vi "2022_day01.vi"() -> ()   [LabVIEW 2021]
uses:
  2f9034f6-0eee-4750-bf2c-0a9c5446afb1.vi
  <vilib>/Comparison/Less/Less Functor/Less Functor.lvclass
panel:
  out "Sum of TOP Calories (task 2)":i32
  in  "Sel. TOP cnt":i32=3
  out "TOP Calories":i32[](array[numeric])
  out "max Calories (task 1)":i32
  out "Raw data":i32[](array[numeric])
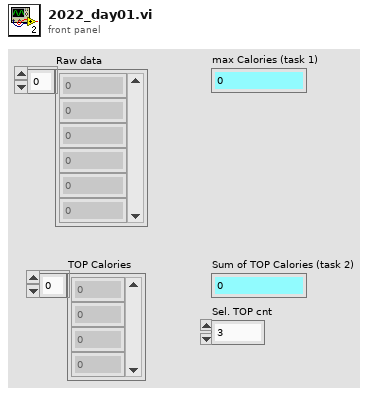
[diagram p1: front panel]
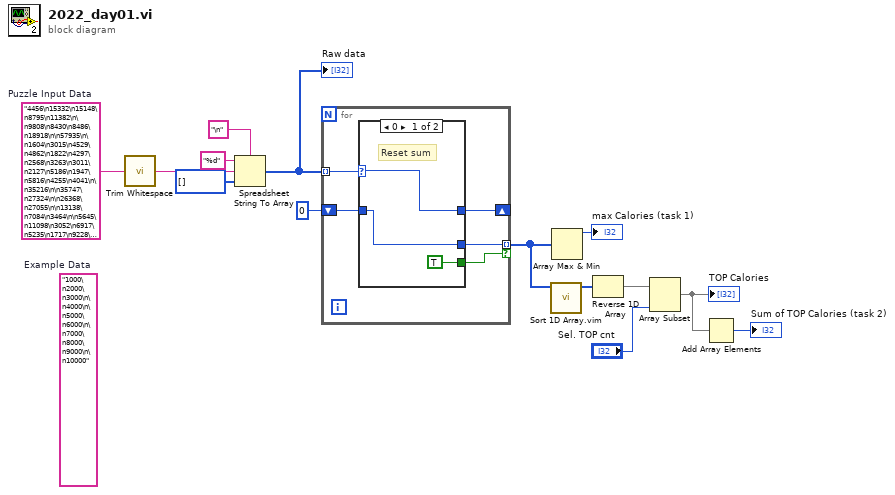
[diagram p0: block diagram]
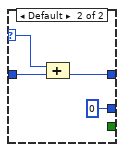
[diagram p2: hidden frame]
diagram:
  (unwired) "1000\n2000\n3000\n\n4000\n\n5000\n6000\n\n7000\n8000\n9000\n\n10000"  # Example Data
  w7 = "4456\n15332\n15148\n8795\n11382\n\n9808\n8430\n8486\n18918\n\n57935\n\n1604\n3015\n4529\n4862\n1822\n4297\n2568\n3263\n3011\n2127\n5186\n1947\n5816\n4255\n4041\n\n35216\n\n35747\n27324\n\n26368\n27055\n\n13138\n7084\n3464\n\n5645\n11098\n3052\n6917\n5235\n1717\n9228\n\n7789\n9290\n5753\n9600\n8631\n6873\n8844\n2228\n5123\n\n5177\n7591\n7973\n2093\n7266\n5307\n3562\n4994\n2681\n2924\n\n15474\n11021\n14987\n18512\n\n12187\n6865\n20315\n\n13751\n\n6467\n8287\n14768\n7194\n9595\n\n3948\n1577\n1989\n\n24800\n23570\n\n2378\n3426\n6782\n7276\n5242\n3067\n4899\n5532\n4877\n6314\n6935\n1956\n\n59761\n\n15344\n4376\n10193\n2616\n4785\n\n2213\n5782\n1524\n5941\n3889\n4619\n5429\n2136\n2728\n3576\n2656\n5164\n4329\n2497\n4708\n\n5683..."  # Puzzle Input Data
  n1 = call <vilib>:"Trim Whitespace.vi"("string"=w7) -> ("trimmed string"=w9:string)  [unwired: 1 in]
  n2 = Spreadsheet String To Array(delimiter (Tab)="\n", format string="%d", spreadsheet string=w9, array type (2D Dbl)=i32[] []) -> (array=w10:i32[])
  "Raw data" <- w10
  n3 = for {
    tunnel: w10 -> [w17] mode=indexing
    shift-right: [w18] -> _
    shift-left: 0 -> [w19]
    tunnel: [w16] -> w6 mode=indexing if=w15
    n4 = case shown="0" w17 {
      selector: w17 -> [w22 w25]
      tunnel: w19 -> [w21 w26]
      tunnel: [w22 w24] -> w18
      tunnel: [w21 0] -> w16
      tunnel: [TRUE _] -> w15
      frame 0 {
        # "Reset sum"
      }
      frame Default {
        n5 = Compound Arithmetic op=ADD(w25, w26) -> (w24:i32)
      }
    }
  }
  n6 = call "Sort 1D Array.vim"("unsorted array"=w6) -> ("sorted array"=w5:i32[])  [unwired: 10 in]
  n7 = Array Max & Min(array=w6) -> (max value=→"max Calories (task 1)":i32)  [unwired: 3 out]
  n8 = Reverse 1D Array(array=w5) -> (reversed array=w4:i32[])
  n9 = Array Subset(array=w4, length="Sel. TOP cnt") -> (w2:i32[])  [unwired: 1 in]
  "TOP Calories" <- w2
  n10 = Add Array Elements(numeric array=w2) -> (sum=→"Sum of TOP Calories (task 2)":i32)
